vi "Merge Rects Verticallyv1.vi"(1 "First":i32[](array[numeric]), 2 "Second":i32[](array[numeric]), 3 "Above":bool) -> (0 "Rect":T1)   [LabVIEW 2013]
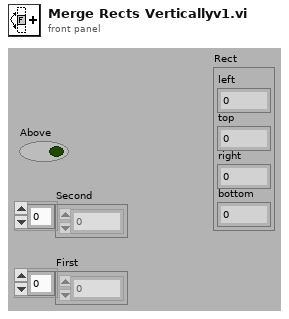
[diagram p1: front panel]
types:
  T1 = cluster{"left":i32, "top":i32, "right":i32, "bottom":i32}
  T2 = cluster{"First[0]":i32, "First[1]":i32, "First[2]":i32, "First[3]":i32}
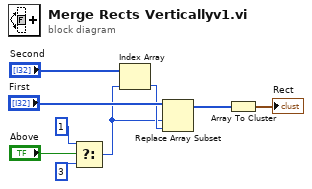
[diagram p0: block diagram]
diagram:
  n1 = Select(t=1, s="Above", f=3) -> (s? t:f=w3:i32)
  n2 = Index Array(array="Second", index=w3) -> (element=w7:i32)
  n3 = Replace Array Subset(array="First", new element=w7, index=w3) -> (w2:i32[])
  n4 = Array To Cluster(array=w2) -> (cluster=→"Rect":T2)
